vi "Meas Result Export - Build Report.vi"(6 "equivalent connection":T3, 8 "error in (no error)":errorcluster, 9 "swp com":string caption="Measurement comment", 10 "append header":bool, 11 "meas":T4={"swp cfg"={"N"=0, "R"=0, "f list"=[], "smpl delay"=0.0, "set delay"=0.0, "set delay np"=0.0, "meas root"=path "", "meas name"="", "meas a-index"=FALSE, "rnd sweep"=FALSE, "mode"=enum."Frequency", "swp mode"=enum."Linear", "avg"=0, "subrec"=0, "multi-freq"=FALSE, "selfcal"=FALSE, "selfcal period [h]"=0.0}, "bridge"={"type"=enum."TWM client", "TWM"={"pipe name"="", "parameters"=[], "handle"=0, "fixed aper [s]"=0.0, "f-list [Hz]"=[], "discrete f-list"=FALSE, "unc mode"=enum."None", "unc mcc"=0, "unc first"=FALSE, "alg id"=enum."TWM-LowZ - Low Z measurement"}, "last f"=0.0, "bias comp"={"bias type"=enum."dummy", "VISA"="", "Enable"=FALSE, "channel qu"=[], "channel Uinit"=[]}, "sim mode"=enum."Generic RLC network", "channel idns"=[], "sim phases"=0}, "src"={"type"=enum."Tektronix AFG3101C", "idn"="", "afg"={"VISA"="", "const"=0.0, "gen DC"=FALSE, "ext ref"=FALSE}, "cDAQ dds"={"device"="", "channels"=[], "mclk source"="", "mclk [Hz]"=0.0, "fs [Hz]"=0.0, "block [s]"=0.0, "buf [s]"=0.0, "task"="", "cmd queue"=refnum, "proc ref"=refnum, "smpl clock out"="", "export smpl clock"=FALSE, "DC ofs [V]"=[], "timebase source"="", "timebase mode"=enum."Local", "dither"=enum."Disabled", "dither level"=0.0, "phase [rad]"=[]}, "gain [V/A]"=0.0, "F5xxx session"={"VISA"="", "mode"=enum."AC voltage", "Earth on"=FALSE, "Ext ref lock"=FALSE}, "t3awg"={"VISA"="", "use ext ref"=FALSE, "ext ref [Hz]"=0.0, "load Z"=enum."High Z", "ramdac max n"=0, "noise dither [V]"=0.0, "t3awg fs rules"=[], "channels"=0, "ramdac min n"=0, "channel list"=[], "gen resl [Vpp]"=0.0, "wave data format"=enum."Binary"}}, "results"=refnum, "dvm"={"type"=enum."Disabled", "idn"="", "F5790"={"VISA"="", "Input"=enum."input 1", "Digital filter restart"=enum."medium", "hi resolution"=enum."off", "Digital filter mode"=enum."off", "ext guard"=FALSE}}, "thermo"={"type"=enum."COMET Tx5xx (ethernet)", "comment"="", "tag"="", "refresh"=5.0, "IP"="", "port"=502, "VISA"="", "last readout"=timestamp(0 s since 1904-01-01), "TCP ref"=refnum, "VISA sess"="", "idn"="", "press"=0.0, "RH"=0.0, "temp"=0.0, "pres cor"=[], "RH cor"=[], "temp cor"=[], "try left"=0, "failed"=FALSE, "RTD set"=[], "RTD inv"=[], "range"=0.0, "net mode"=enum."MODBUS", "try fail"=enum."Stop trying - return NaN", "timeout [s]"=0.0, "max retries"=0, "sim t [deg]"=0.0, "status"=0}} {"thermo"."status" items=["ok", "retry", "failed"]; "thermo"."RTD inv" format="%.1f"; "thermo"."RTD set" format="%.1f"; "thermo"."temp cor" format="%.1f"; "thermo"."RH cor" format="%.1f"; "thermo"."pres cor" format="%.1f"; "thermo"."refresh" min=0.1 max=1000.0 format="%.2f"; "src"."t3awg"."t3awg fs rules"."fs-step [Hz]" format="%#_6p"; "src"."t3awg"."t3awg fs rules"."fs-max [Hz]" format="%#_6p"; "src"."t3awg"."t3awg fs rules"."for f0 <" format="%#_6p"; "src"."t3awg"."t3awg fs rules"."fs-min [Hz]" format="%#_6p"; "src"."cDAQ dds"."channels" min=0 step=1; "bridge"."TWM"."f-list [Hz]" format="%#_6p"; "swp cfg"."f list"."bias" format="%#_3p"; "swp cfg"."f list"."level" format="%#_3p"; "swp cfg"."f list"."fs [Hz]" format="%#_5p"; "swp cfg"."f list"."time [s]" format="%#_3p"; "swp cfg"."f list"."f/fs" format="%#_3p"; "swp cfg"."f list"."periods" format="%#_3f"; "swp cfg"."f list"."f [Hz]" format="%#_5p"}) -> (0 "error out":errorcluster, 3 "report":string[][](array[string]))   [LabVIEW 2020]
doc: "Generates simple results report in form of text matrix."
uses:
  meas session.ctl
  Meas Sweep Config.ctl
  Meas Freq Info.ctl
  meas_swp_mode.ctl
  meas_sweep_flist_mode.ctl
  bridge/Bridge Session.ctl
  bridge/Bridge Type.ctl
  drivers/TWM client/TWM Session.ctl
  drivers/TWM client/TWM parameters.ctl
  drivers/TWM client/Meas Proc QWTB Uncertainty Mode.ctl
  bridge/Bridge Algorithm.ctl
  bridge/Bridge Bias Session.ctl
  bridge/Bridge Bias Type.ctl
  bridge/Bridge Sim Mode.ctl
  source/Source Session.ctl
  source/Source Type.ctl
  drivers/AFG3101C/AFG3101C Session.ctl
  drivers/cDAQ DDS/cDAQ DDS Session.ctl
  drivers/cDAQ DDS/cDAQ DDS Setup.ctl
  drivers/cDAQ DDS/cDAQ DDS Timebase Mode.ctl
  drivers/cDAQ DDS/cDAQ DDS Dither.ctl
  drivers/Fluke 5XXX/top_lev/F5xxx_session.ctl
  drivers/Fluke 5XXX/top_lev/F5xxx_output_mode.ctl
  drivers/T3AWG3K/toplevel/T3AWG Session.ctl
  drivers/T3AWG3K/toplevel/T3AWG Load Z.ctl
  drivers/T3AWG3K/toplevel/fgen_ramdac_fs_rules.ctl
  drivers/T3AWG3K/toplevel/T3AWG Channel.ctl
  Meas Results Ref.ctl
  Meas Results.ctl
  bridge/Bridge Frequency Readings Data.ctl
  drivers/TWM client/Meas Proc QWTB Spectrum Data.ctl
  drivers/TWM client/TWM Phase Info.ctl
  dvm/dvm session.ctl
  dvm/dvm type.ctl
  drivers/Fluke 5790A/top_level/F5790 session.ctl
  thermo/thermo.ctl
  thermo/thermo_types.ctl
  thermo/Thermometer Fail Action.ctl
  Impedance Equivalent Circuit.ctl
  Meas Results Sweep Data Uncertainty Mode.ctl
  varilib/varilib.lvlib
  drivers/T3AWG3K/Active Technologies AWG3000.lvlib
panel:
  in  "dvm type":T1
  in  "thermo type":T2 caption="type"
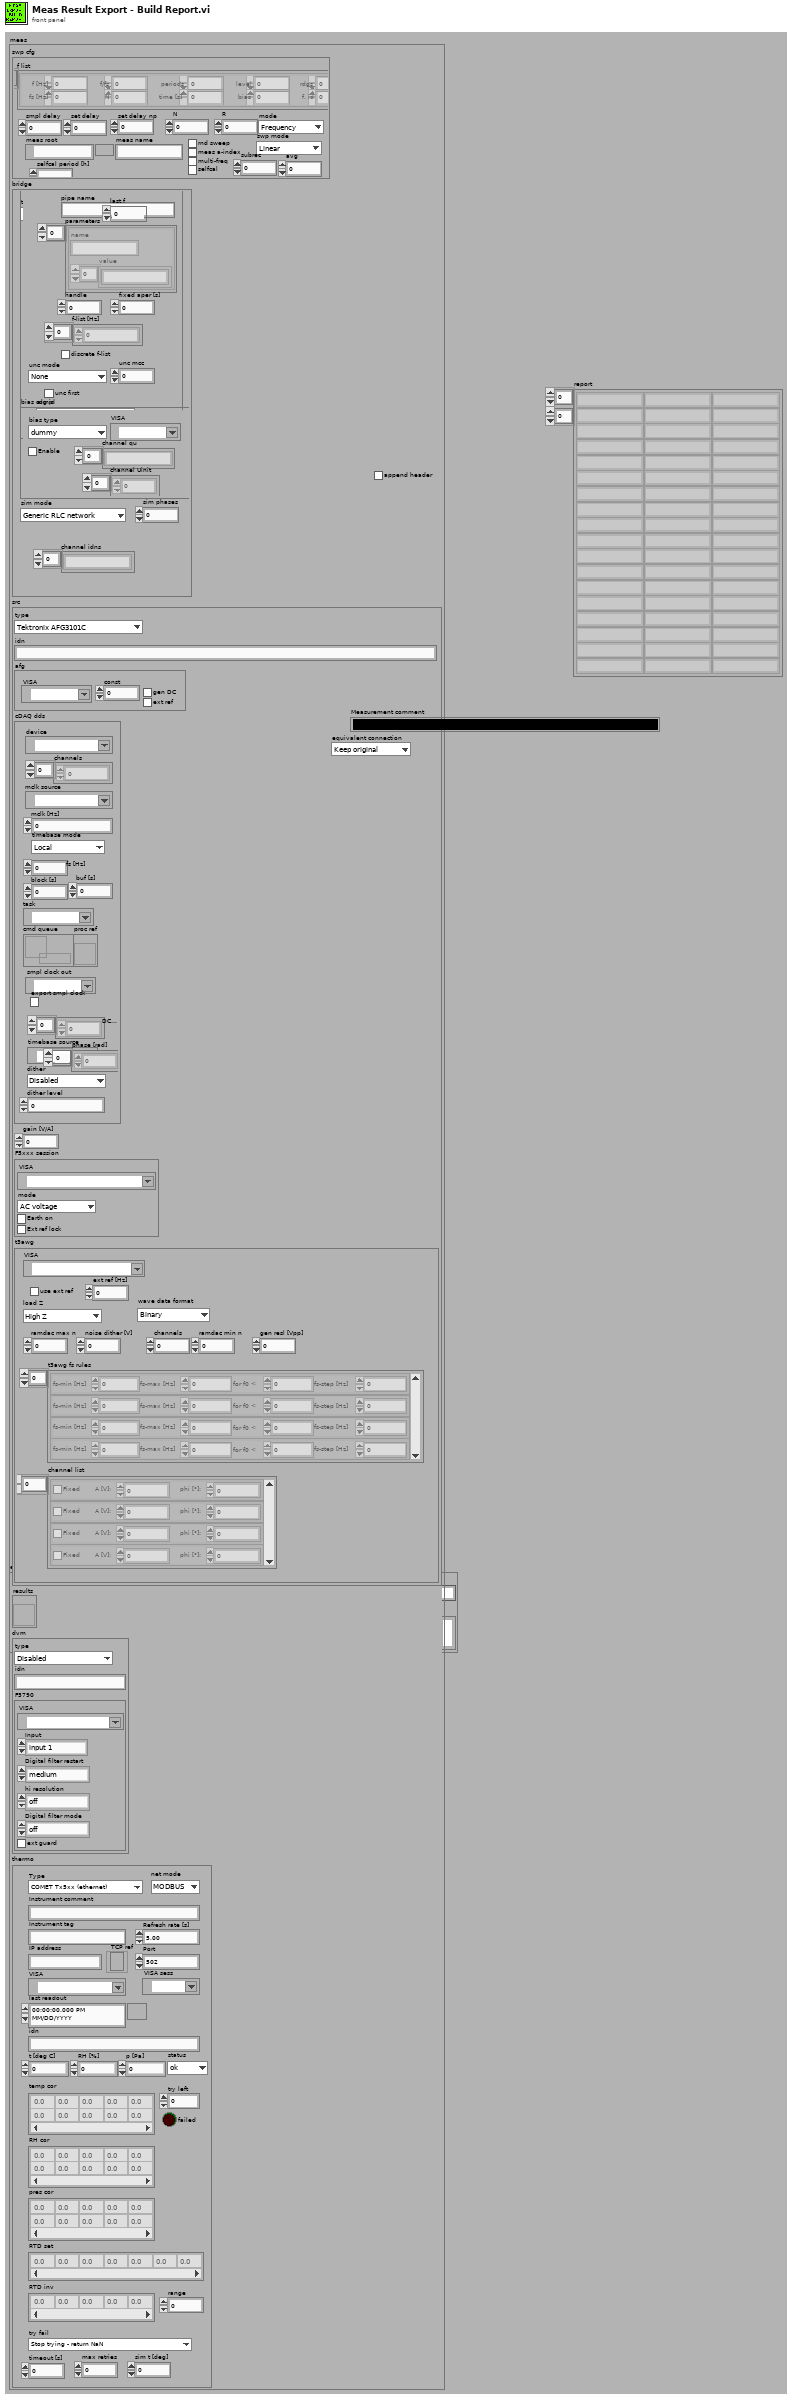
[diagram p1: front panel]
types:
  T1 = typedef "dvm type.ctl" = enum16{"Disabled", "Simulated", "Fluke 5790A"}
  T2 = typedef "thermo_types.ctl" = enum16{"Disabled", "Simulated", "COMET Tx5xx (ethernet)", "Keithley 2002 (GPIB) + RTD", "Agilent 344xx (GPIB) + RTD"}
  T3 = typedef "Impedance Equivalent Circuit.ctl" = enum16{"Keep original", "Rs-Xs", "Gp-Bp", "Z-phid", "Z-phir", "Y-phid", "Y-phir", "Cp-D", "Cp-Q", "Cp-Rp", "Cp-Gp", "Cs-D", "Cs-Q", "Cs-Rs", "Ls-Rs", "Ls-Q", "Rs-Tau"}
  T4 = typedef "meas session.ctl" = cluster{"swp cfg":T5, "bridge":T9, "src":T18, "results":T31, "dvm":T32, "thermo":T34}
  T5 = typedef "Meas Sweep Config.ctl" = cluster{"N":i32, "R":i32, "f list":T6[], "smpl delay":dbl, "set delay":dbl, "set delay np":dbl, "meas root":path, "meas name":string, "meas a-index":bool, "rnd sweep":bool, "mode":T7, "swp mode":T8, "avg":i32, "subrec":i32, "multi-freq":bool, "selfcal":bool, "selfcal period [h]":dbl}
  T6 = typedef "Meas Freq Info.ctl" = cluster{"f [Hz]":dbl, "periods":dbl, "f/fs":dbl, "time [s]":dbl, "fs [Hz]":dbl, "N":i32, "level":dbl, "bias":dbl, "rdgs":i32, "f. id":i32}
  T7 = typedef "meas_swp_mode.ctl" = enum16{"Frequency", "Level", "Bias"}
  T8 = typedef "meas_sweep_flist_mode.ctl" = enum16{"Linear", "Log10"}
  T9 = typedef "Bridge Session.ctl" = cluster{"type":T10, "TWM":T11, "last f":dbl, "bias comp":T15, "sim mode":T17, "channel idns":string[], "sim phases":i32}
  T10 = typedef "Bridge Type.ctl" = enum16{"TWM client", "dummy"}
  T11 = typedef "TWM Session.ctl" = cluster{"pipe name":string, "parameters":T12[], "handle":i32, "fixed aper [s]":dbl, "f-list [Hz]":dbl[], "discrete f-list":bool, "unc mode":T13, "unc mcc":i32, "unc first":bool, "alg id":T14}
  T12 = typedef "TWM parameters.ctl" = cluster{"name":string, "value":string[]}
  T13 = typedef "Meas Proc QWTB Uncertainty Mode.ctl" = enum16{"None", "GUF", "Monte Carlo"}
  T14 = typedef "Bridge Algorithm.ctl" = enum16{"TWM-LowZ - Low Z measurement", "TWM-InpZ - Digitizer input Z measurement", "TWM-TIAZ - High Z using TIA"}
  T15 = typedef "Bridge Bias Session.ctl" = cluster{"bias type":T16, "VISA":refnum<visa-resource-name>, "Enable":bool, "channel qu":string[], "channel Uinit":dbl[]}
  T16 = typedef "Bridge Bias Type.ctl" = enum16{"dummy", "CMI LiBbias V1.0"}
  T17 = typedef "Bridge Sim Mode.ctl" = enum16{"Generic RLC network", "Interchannel transfer", "Input impedance"}
  T18 = typedef "Source Session.ctl" = cluster{"type":T19, "idn":string, "afg":T20, "cDAQ dds":T21, "gain [V/A]":dbl, "F5xxx session":T24, "t3awg":T26}
  T19 = typedef "Source Type.ctl" = enum16{"Tektronix AFG3101C", "cDAQ DAC", "Fluke 5xxx", "Agilent 33120A", "R&S SMT", "Teledyne LeCroy T3AWG", "dummy"}
  T20 = typedef "AFG3101C Session.ctl" = cluster{"VISA":refnum<visa-resource-name>, "const":dbl, "gen DC":bool, "ext ref":bool}
  T21 = typedef "cDAQ DDS Session.ctl" = cluster{"device":tag, "channels":i32[], "mclk source":tag, "mclk [Hz]":dbl, "fs [Hz]":dbl, "block [s]":dbl, "buf [s]":dbl, "task":refnum<k21>, "cmd queue":refnum<queue>, "proc ref":refnum<vi>, "smpl clock out":tag, "export smpl clock":bool, "DC ofs [V]":dbl[], "timebase source":tag, "timebase mode":T22, "dither":T23, "dither level":dbl, "phase [rad]":dbl[]}
  T22 = typedef "cDAQ DDS Timebase Mode.ctl" = enum16{"Local", "Take from ADC (e.g. NI 9238)", "Other source"}
  T23 = typedef "cDAQ DDS Dither.ctl" = enum16{"Disabled", "Gaussian"}
  T24 = typedef "F5xxx_session.ctl" = cluster{"VISA":refnum<visa-resource-name>, "mode":T25, "Earth on":bool, "Ext ref lock":bool}
  T25 = typedef "F5xxx_output_mode.ctl" = enum16{"AC voltage", "AC current"}
  T26 = typedef "Active Technologies AWG3000.lvlib/T3AWG Session.ctl" = cluster{"VISA":refnum<visa-resource-name>, "use ext ref":bool, "ext ref [Hz]":dbl, "load Z":T27, "ramdac max n":i32, "noise dither [V]":dbl, "t3awg fs rules":T28[], "channels":i32, "ramdac min n":i32, "channel list":T29[], "gen resl [Vpp]":dbl, "wave data format":T30}
  T27 = typedef "Active Technologies AWG3000.lvlib/T3AWG Load Z.ctl" = enum16{"High Z", "50 Ohm"}
  T28 = typedef "Active Technologies AWG3000.lvlib/fgen_ramdac_fs_rules.ctl" = cluster{"fs-min [Hz]":dbl, "fs-max [Hz]":dbl, "for f0 < ":dbl, "fs-step [Hz]":dbl}
  T29 = typedef "Active Technologies AWG3000.lvlib/T3AWG Channel.ctl" = cluster{"Fixed":bool, "A [V]:":dbl, "phi [°]:":dbl}
  T30 = typedef "Active Technologies AWG3000.lvlib/T3AWG Wave Format" = enum16{"Text", "Binary"}
  T31 = typedef "Meas Results Ref.ctl" = refnum<vi>
  T32 = typedef "dvm session.ctl" = cluster{"type":T1, "idn":string, "F5790":T33}
  T33 = typedef "F5790 session.ctl" = cluster{"VISA":refnum<visa-resource-name>, "Input":enum16{"input 1", "input 2", "wide-band"}, "Digital filter restart":enum16{"medium", "fine", "coarse"}, "hi resolution":enum16{"off", "on"}, "Digital filter mode":enum16{"off", "fast", "medium", "slow"}, "ext guard":bool}
  T34 = typedef "thermo.ctl" = cluster{"type":T2, "comment":string, "tag":string, "refresh":dbl, "IP":string, "port":u16, "VISA":refnum<visa-resource-name>, "last readout":timestamp, "TCP ref":refnum<k5>, "VISA sess":refnum<visa-resource-name>, "idn":string, "press":dbl, "RH":dbl, "temp":dbl, "pres cor":dbl[][], "RH cor":dbl[][], "temp cor":dbl[][], "try left":i32, "failed":bool, "RTD set":dbl[], "RTD inv":dbl[], "range":dbl, "net mode":enum16{"MODBUS", "HTTP"}, "try fail":T35, "timeout [s]":dbl, "max retries":i32, "sim t [deg]":dbl, "status":u16}
  T35 = typedef "Thermometer Fail Action.ctl" = enum16{"Stop trying - keep last value", "Stop trying - return NaN", "Generate error - stop sweep"}
  T36 = typedef "Meas Results Sweep Data Uncertainty Mode.ctl" = enum16{"ua(y)", "ua(y) (p=95%)", "uc(y) (p=95%)"}
  T37 = typedef "Meas Results.ctl" = cluster{"freqs":T38[][], "locked":bool, "last fid":i32, "modified":bool, "mjr name":string, "mnr name":string, "last spectra":T39[][], "saved?":bool, "TWM phase":T40[], "time start":timestamp, "time stop":timestamp, "equ cct":string}
  T38 = typedef "Bridge Frequency Readings Data.ctl" = cluster{"Udut":dbl[], "Iref":dbl[], "Udc":dbl[], "Idc":dbl[], "mjr":dbl[], "mnr":dbl[], "mjr_sh":dbl[], "mnr_sh":dbl[], "u(mjr)":dbl[], "u(mnr)":dbl[], "ua2(mjr)":dbl[], "ua2(mnr)":dbl[], "n":i32, "f [Hz]":dbl, "fs [Hz]":dbl, "aperture [s]":dbl, "Udvm":dbl[], "u(Udvm) [V]":dbl, "t_dut [degC]":dbl[], "RH_dut [%]":dbl[], "p_dut [Pa]":dbl[], "timestamp":timestamp[], "level":dbl, "bias":dbl}
  T39 = typedef "Meas Proc QWTB Spectrum Data.ctl" = cluster{"x":sgl[], "y":sgl[], "label":string}
  T40 = typedef "TWM Phase Info.ctl" = cluster{"ref chn id (I)":string, "dut chn id (U)":string, "ref chn range [V]":dbl, "dut chn range [V]":dbl, "aperture [s]":dbl, "fs [Hz]":dbl, "ref chn transducer (I)":string, "dut chn transducer (U)":string}
  T41 = typedef "Meas Results Sweep Data.ctl" = cluster{"Udut":dbl[], "Iref":dbl[], "Udc":dbl[], "Idc":dbl[], "mjr":dbl[], "mnr":dbl[], "mjr_sh":dbl[], "mnr_sh":dbl[], "f [Hz]":dbl[], "n [-]":i32[], "fs [Hz]":dbl[], "aperture [s]":dbl[], "Udvm":dbl[], "t_dut [degC]":dbl[], "RH_dut [%]":dbl[], "p_dut [Pa]":dbl[], "level":dbl[], "bias":dbl[]}
  T42 = typedef "Meas Quantity Names.ctl" = cluster{"mjr name":string, "mnr name":string, "mjr unit":string, "mnr unit":string, "mjr full":string, "mnr full":string}
  T43 = typedef "Source Info.ctl" = cluster{"type":string, "address":string, "idn":string, "aux headers":string[], "aux data":string[]}
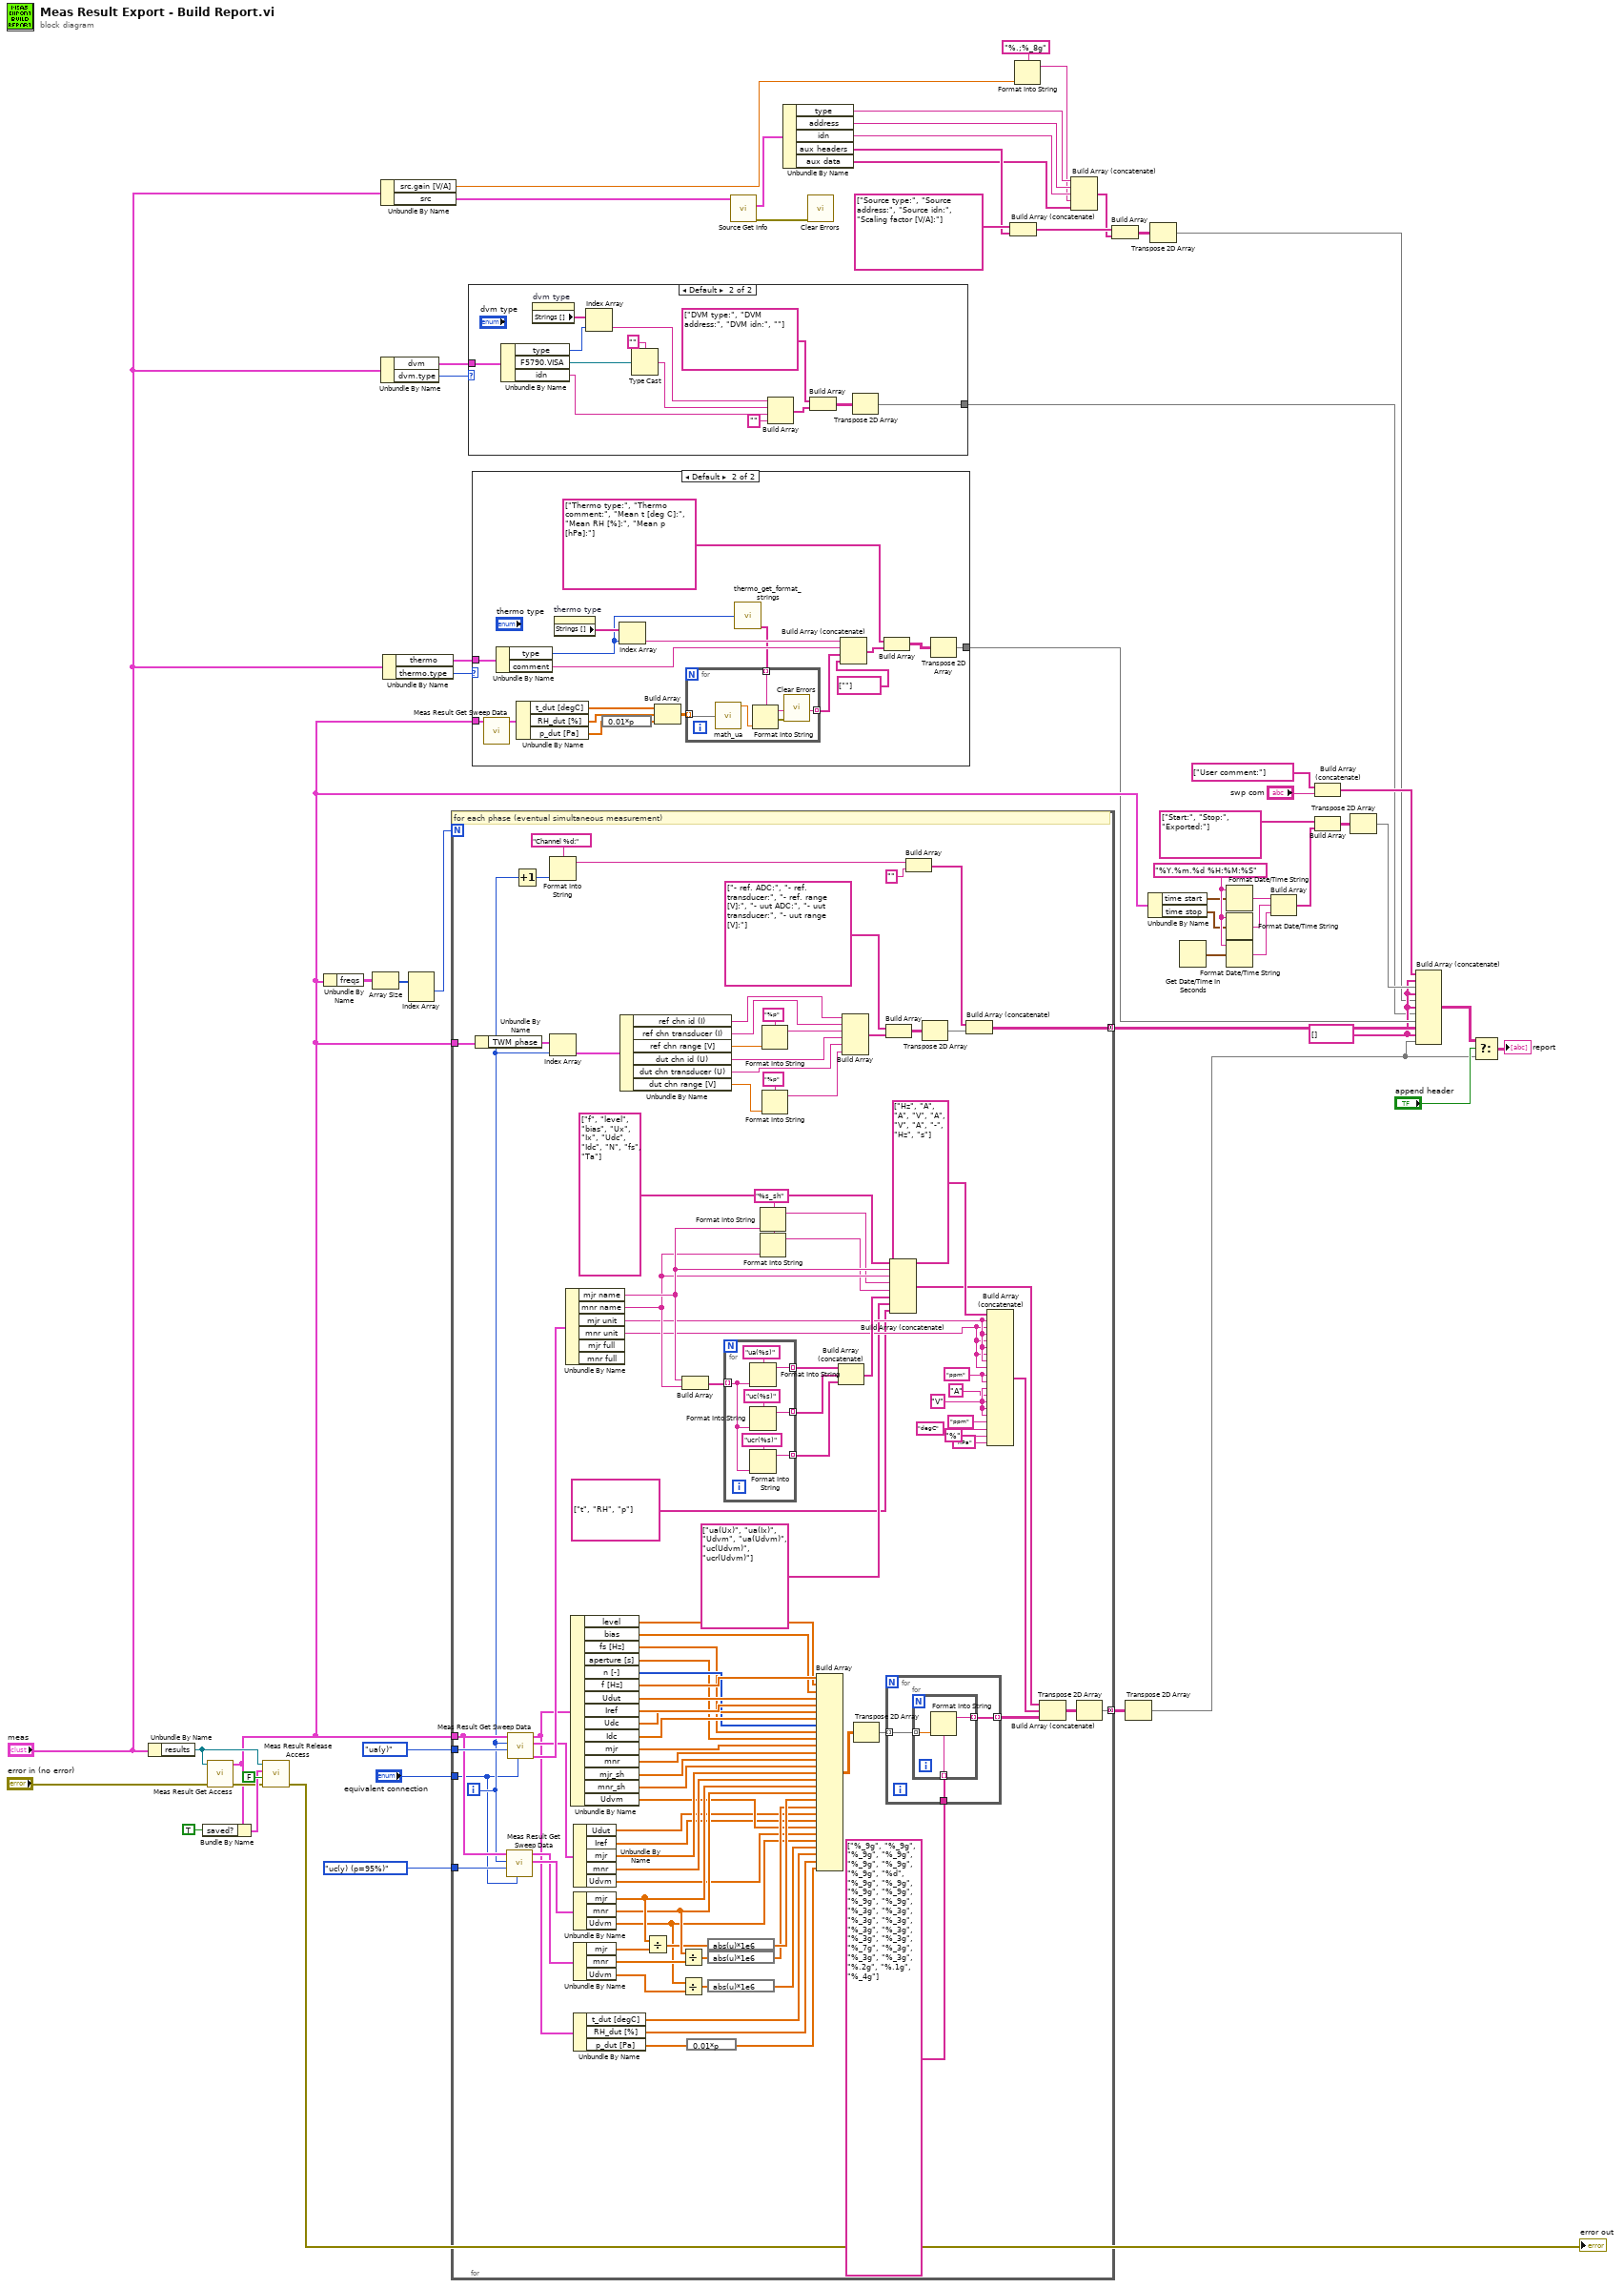
[diagram p0: block diagram]
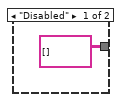
[diagram p2: hidden frame]
diagram:
  w16 = string[] [] ("array")
  w35 = "%Y.%m.%d %H:%M:%S" ("format string")
  n1 = Unbundle By Name("meas") -> ("results"=w53:T31)
  n2 = call "Meas Result Get Access.vi"("error in"="error in (no error)", "results ref"=w53) -> ("error out"=w50:errorcluster, "results data"=w23:T37)  [unwired: 8 in]
  n3 = Bundle By Name(cluster=w23, "saved?"=TRUE) -> (w52:T37)
  n4 = call "Meas Result Release Access.vi"("error in"=w50, "Release only (True)"=FALSE, "results data in"=w52, "results ref"=w53) -> ("error out"=→"error out":errorcluster)  [unwired: 7 in]
  n5 = Unbundle By Name(w23) -> ("freqs"=w47:T38[][])
  n6 = Array Size(array=w47) -> (size(s)=w48:i32[])
  n7 = Unbundle By Name("meas") -> ("src.gain [V/A]"=w2:dbl, "src"=w19:T18)
  n8 = Unbundle By Name("meas") -> ("dvm"=w20:T32, "dvm.type"=w21:T1)
  n9 = Unbundle By Name("meas") -> ("thermo"=w24:T34, "thermo.type"=w25:T2)
  n10 = Index Array(array=w48) -> (element #1=w49:i32)  [unwired: 2 in, 1 out]
  n11 = for {
    N: w49 -> [_]
    tunnel: [w111] -> w44 mode=concatenating
    tunnel: Meas_Results_Sweep_Data_Uncertainty_Mode."ua(y)" ("uncertainty mode") -> [w141]
    tunnel: w23 -> [w140]
    tunnel: Meas_Results_Sweep_Data_Uncertainty_Mode."uc(y) (p=95%)" ("uncertainty mode") -> [w139]
    tunnel: w23 -> [w109]
    tunnel: [w86] -> w58 mode=concatenating
    tunnel: "equivalent connection" -> [w76]
    i -> [w105]
    w65 = "V" ("element")
    w113 = "ppm" ("element")
    w129 = "%s_sh" ("format string")
    # "for each phase (eventual simultaneous measurement)"
    n12 = Unbundle By Name(w109) -> ("TWM phase"=w108:T40[])
    n13 = call "Meas Result Get Sweep Data.vi"("equ connection override"=w76, "uncertainty mode"=w139, "phase index (default: 0)"=w105, "result"=w140) -> ("unc(data)"=w138:T41, "data"=w122:T41)  [unwired: 5 in, 1 out]
    n14 = call "Meas Result Get Sweep Data.vi"("equ connection override"=w76, "uncertainty mode"=w141, "phase index (default: 0)"=w105, "result"=w140) -> ("quantities"=w158:T42, "unc(data)"=w71:T41, "data"=w67:T41)  [unwired: 5 in]
    n15 = Increment(x=w105) -> (x+1=w104:i32)
    n16 = Format Into String(format string="Channel %d:", w104) -> (resulting string=w103:string)  [unwired: 2 in, 1 out]
    n17 = Index Array(array=w108, index=w105) -> (element=w107:T40)
    n18 = Unbundle By Name(w158) -> ("mjr name"=w128:string, "mnr name"=w127:string, "mjr unit"=w124:string, "mnr unit"=w123:string)  [unwired: 2 out]
    n19 = Unbundle By Name(w67) -> ("level"=w60:dbl[], "bias"=w59:dbl[], "fs [Hz]"=w78:dbl[], "aperture [s]"=w77:dbl[], "n [-]"=w110:i32[], "f [Hz]"=w156:dbl[], "Udut"=w155:dbl[], "Iref"=w154:dbl[], "Udc"=w153:dbl[], "Idc"=w152:dbl[], "mjr"=w151:dbl[], "mnr"=w150:dbl[], "mjr_sh"=w131:dbl[], "mnr_sh"=w130:dbl[], "Udvm"=w63:dbl[])
    n20 = Unbundle By Name(w71) -> ("Udut"=w62:dbl[], "Iref"=w61:dbl[], "mjr"=w137:dbl[], "mnr"=w136:dbl[], "Udvm"=w83:dbl[])
    n21 = Unbundle By Name(w138) -> ("mjr"=w121:dbl[], "mnr"=w118:dbl[], "Udvm"=w80:dbl[])
    n22 = Unbundle By Name(w122) -> ("mjr"=w120:dbl[], "mnr"=w119:dbl[], "Udvm"=w81:dbl[])
    n23 = Unbundle By Name(w67) -> ("t_dut [degC]"=w70:dbl[], "RH_dut [%]"=w69:dbl[], "p_dut [Pa]"=w68:dbl[])
    n24 = Unbundle By Name(w107) -> ("ref chn id (I)"=w95:string, "ref chn transducer (I)"=w96:string, "ref chn range [V]"=w101:dbl, "dut chn id (U)"=w94:string, "dut chn transducer (U)"=w93:string, "dut chn range [V]"=w98:dbl)
    n25 = Divide(x=w121, y=w120) -> (x/y=w116:dbl[])
    n26 = Divide(x=w118, y=w119) -> (x/y=w117:dbl[])
    n27 = Divide(x=w80, y=w81) -> (x/y=w82:dbl[])
    n28 = Build Array(w128, w127) -> (w135:string[])
    n29 = expression code="0.01*p"(w68) -> (w66:dbl[])
    n30 = expression code="abs(u)*1e6"(w116) -> (w115:dbl[])
    n31 = expression code="abs(u)*1e6"(w117) -> (w114:dbl[])
    n32 = expression code="abs(u)*1e6"(w82) -> (w79:dbl[])
    n33 = for {
      tunnel: w135 -> [w160] mode=indexing
      tunnel: [w163] -> w134 mode=indexing
      tunnel: [w162] -> w133 mode=indexing
      tunnel: [w159] -> w112 mode=indexing
      n34 = Format Into String(format string="ua(%s)", w160) -> (resulting string=w163:string)  [unwired: 2 in, 1 out]
      n35 = Format Into String(format string="uc(%s)", w160) -> (resulting string=w162:string)  [unwired: 2 in, 1 out]
      n36 = Format Into String(format string="ucr(%s)", w160) -> (resulting string=w159:string)  [unwired: 2 in, 1 out]
    }
    n37 = Format Into String(format string=w129, w128) -> (resulting string=w126:string)  [unwired: 2 in, 1 out]
    n38 = Format Into String(format string=w129, w127) -> (resulting string=w125:string)  [unwired: 2 in, 1 out]
    n39 = Format Into String(format string="%p", w101) -> (resulting string=w97:string)  [unwired: 2 in, 1 out]
    n40 = Format Into String(format string="%p", w98) -> (resulting string=w92:string)  [unwired: 2 in, 1 out]
    n41 = Build Array(w156, w60, w59, w155, w154, w153, w152, w110, w78, w77, w151, w150, w131, w130, w137, w136, w121, w118, w115, w114, w62, w61, w63, w83, w80, w79, w70, w69, w66) -> (w148:dbl[][])
    n42 = Build Array (concatenate)(w134, w133, w112) -> (w132:string[])
    n43 = Build Array(w95, w96, w97, w94, w93, w92) -> (w91:string[])
    n44 = Transpose 2D Array(2D array=w148) -> (transposed array=w147:dbl[][])
    n45 = Build Array(string[] ["- ref. ADC:", "- ref. transducer:", "- ref. range [V]:", "- uut ADC:", "- uut transducer:", "- uut range [V]:"], w91) -> (w89:string[][])
    n46 = for {
      tunnel: w147 -> [w167] mode=indexing
      tunnel: string[] ["%_9g", "%_9g", "%_9g", "%_9g", "%_9g", "%_9g", "%_9g", "%d", "%_9g", "%_9g", "%_9g", "%_9g", "%_9g", "%_9g", "%_3g", "%_3g", "%_3g", "%_3g", "%_3g", "%_3g", "%_3g", "%_3g", "%_7g", "%_3g", "%_3g", "%_3g", "%.2g", "%.1g", "%_4g"] -> [w168]
      tunnel: [w166] -> w145 mode=indexing
      n47 = for {
        tunnel: w168 -> [w170] mode=indexing
        tunnel: w167 -> [w171] mode=indexing
        tunnel: [w169] -> w166 mode=indexing
        n48 = Format Into String(format string=w170, w171) -> (resulting string=w169:string)  [unwired: 2 in, 1 out]
      }
    }
    n49 = Build Array (concatenate)(string[] ["f", "level", "bias", "Ux", "Ix", "Udc", "Idc", "N", "fs", "Ta"], w128, w127, w126, w125, w132, string[] ["ua(Ux)", "ua(Ix)", "Udvm", "ua(Udvm)", "uc(Udvm)", "ucr(Udvm)"], string[] ["t", "RH", "p"]) -> (w144:string[])
    n50 = Build Array(w103, "" ("element")) -> (w87:string[])
    n51 = Transpose 2D Array(2D array=w89) -> (transposed array=w88:string[][])
    n52 = Build Array (concatenate)(w87, w88) -> (w86:string[][])
    n53 = Build Array (concatenate)(string[] ["Hz", "A", "A", "V", "A", "V", "A", "-", "Hz", "s"], w124, w123, w124, w123, w124, w123, w124, w123, w113, w113, w65, "A" ("element"), w65, w65, w65, "ppm" ("element"), "degC" ("element"), "%" ("element"), "hPa" ("element")) -> (w143:string[])
    n54 = Build Array (concatenate)(w144, w143, w145) -> (w142:string[][])
    n55 = Transpose 2D Array(2D array=w142) -> (transposed array=w111:string[][])
  }
  n56 = case shown="Default" w21 {
    tunnel: w20 -> [_ w185]
    tunnel: [string[][] [] w174] -> w4
    frame "Disabled" {
    }
    frame Default {
      n57 = Unbundle By Name(w185) -> ("type"=w183:T1, "F5790.VISA"=w182:refnum<visa-resource-name>, "idn"=w175:string)
      n58 = property on="dvm type" class="Enum (strict)"() -> ("Strings []"=w184:string[])  [unwired: 2 in, 2 out]
      n59 = Index Array(array=w184, index=w183) -> (element=w177:string)
      n60 = Type Cast(type="", x=w182) -> (*(type *) &x=w176:string)
      n61 = Build Array(w177, w176, w175, "" ("element")) -> (w178:string[])
      n62 = Build Array(string[] ["DVM type:", "DVM address:", "DVM idn:", ""], w178) -> (w180:string[][])
      n63 = Transpose 2D Array(2D array=w180) -> (transposed array=w174:string[][])
    }
  }
  n64 = case shown="Default" w25 {
    tunnel: w24 -> [_ w204]
    tunnel: w23 -> [_ w200]
    tunnel: [_ w190] -> w22
    frame "Disabled" {
    }
    frame Default {
      n65 = call "Meas Result Get Sweep Data.vi"("result"=w200) -> ("data"=w199:T41)  [unwired: 8 in, 2 out]
      n66 = Unbundle By Name(w204) -> ("type"=w187:T2, "comment"=w201:string)
      n67 = Unbundle By Name(w199) -> ("t_dut [degC]"=w198:dbl[], "RH_dut [%]"=w197:dbl[], "p_dut [Pa]"=w196:dbl[])
      n68 = property on="thermo type" class="Enum (strict)"() -> ("Strings []"=w203:string[])  [unwired: 2 in, 2 out]
      n69 = expression code="0.01*p"(w196) -> (w186:dbl[])
      n70 = Index Array(array=w203, index=w187) -> (element=w202:string)
      n71 = Build Array(w198, w197, w186) -> (w195:dbl[][])
      n72 = call "thermo_get_format_strings.vi"("type index"=w187) -> ("format strings"=w188:string[])  [unwired: 1 in, 3 out]
      n73 = for {
        tunnel: w195 -> [w209] mode=indexing
        tunnel: w188 -> [w207] mode=indexing
        tunnel: [w206] -> w194 mode=indexing
        n74 = call "math_ua.vi"("x"=w209) -> ("mean(x)"=w208:dbl)  [unwired: 3 out]
        n75 = Format Into String(format string=w207, w208) -> (resulting string=w206:string, error out=w205:errorcluster)  [unwired: 2 in]
        n76 = call <vilib>:"Clear Errors.vi"("error in (no error)"=w205) -> ()  [unwired: 5 in, 2 out]
      }
      n77 = Build Array (concatenate)(w202, w201, w194, string[] [""] ("array")) -> (w193:string[])
      n78 = Build Array(string[] ["Thermo type:", "Thermo comment:", "Mean t [deg C]:", "Mean RH [%]:", "Mean p [hPa]:"], w193) -> (w191:string[][])
      n79 = Transpose 2D Array(2D array=w191) -> (transposed array=w190:string[][])
    }
  }
  n80 = call "Source Get Info.vi"("src in"=w19) -> ("error out"=w17:errorcluster, "config info"=w15:T43)  [unwired: 8 in, 1 out]
  n81 = Unbundle By Name(w15) -> ("type"=w12:string, "address"=w11:string, "idn"=w10:string, "aux headers"=w13:string[], "aux data"=w9:string[])
  n82 = call <vilib>:"Clear Errors.vi"("error in (no error)"=w17) -> ()  [unwired: 5 in, 2 out]
  n83 = Build Array (concatenate)(string[] ["Source type:", "Source address:", "Source idn:", "Scaling factor [V/A]:"], w13) -> (w8:string[])
  n84 = Format Into String(format string="%.;%_8g", w2) -> (resulting string=w1:string)  [unwired: 2 in, 1 out]
  n85 = Build Array (concatenate)(w12, w11, w10, w1, w9) -> (w7:string[])
  n86 = Build Array(w8, w7) -> (w6:string[][])
  n87 = Transpose 2D Array(2D array=w44) -> (transposed array=w41:string[][])
  n88 = Unbundle By Name(w23) -> ("time start"=w30:timestamp, "time stop"=w29:timestamp)
  n89 = Transpose 2D Array(2D array=w6) -> (transposed array=w5:string[][])
  n90 = Get Date/Time In Seconds() -> (seconds since 1Jan1904=w36:timestamp)
  n91 = Format Date/Time String(time format string (%c)=w35, seconds (now)=w30) -> (date/time string=w34:string)  [unwired: 1 in]
  n92 = Format Date/Time String(time format string (%c)=w35, seconds (now)=w29) -> (date/time string=w33:string)  [unwired: 1 in]
  n93 = Format Date/Time String(time format string (%c)=w35, seconds (now)=w36) -> (date/time string=w32:string)  [unwired: 1 in]
  n94 = Build Array(w34, w33, w32) -> (w31:string[])
  n95 = Build Array (concatenate)(string[] ["User comment:"], "swp com") -> (w37:string[])
  n96 = Build Array(string[] ["Start:", "Stop:", "Exported:"], w31) -> (w27:string[][])
  n97 = Transpose 2D Array(2D array=w27) -> (transposed array=w28:string[][])
  n98 = Build Array (concatenate)(w37, w16, w28, w16, w5, w16, w4, w22, w58, w16, w41) -> (w43:string[][])
  n99 = Select(t=w43, s="append header", f=w41) -> (s? t:f=→"report":string[][])
